vi "C-885 Test Panel.vi"() -> ()   [LabVIEW 2016]
uses:
  PI GCS2 DLL/PI_GCS2_DLL_x64.dll
panel:
  in  "Set Point":dbl=0.1 format="%#_13g"
  out "Success":u32
  in  "stop":bool
  out "Positions 2":dbl[](array[numeric])
  out "Positions":dbl[](array[numeric])
  out "On Target?":u32[](array[numeric])
  out "Axes Refed":u32[](array[numeric])
  out "Axes ON?":u32[](array[numeric])
  in  "Axes":string[](array[string])
  out "USB Connection Error":bool
  out "C-885 Found":bool
  out "Number Connected":i32
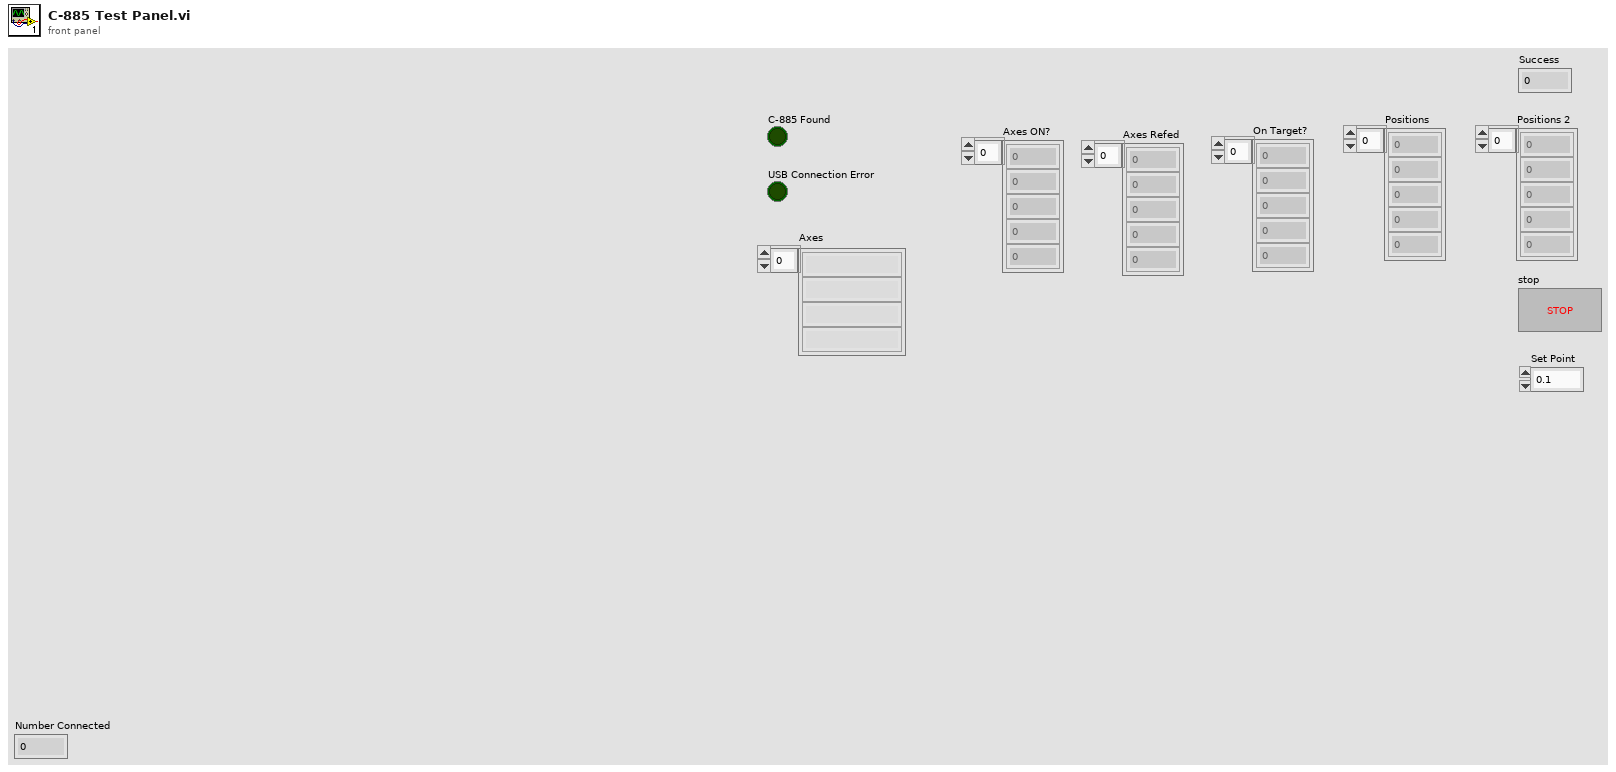
[diagram p1: front panel]
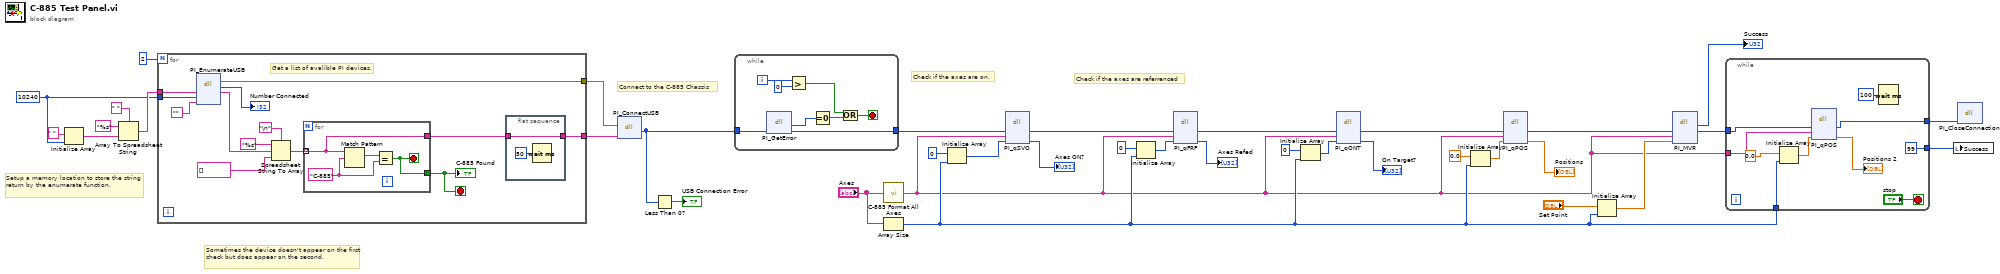
[diagram p0: block diagram]
diagram:
  w32 = 10240 ("dimension size")
  # "Check if the axes are referrenced"
  # "Check if the axes are on."
  # "Setup a memory location to store the string return by the enumerate function."
  # "Connect to the C-885 Chassis"
  # "Sometimes the device doesn't appear on the first check but does appear on the second."
  n1 = Initialize Array(" ", w32) -> (w36:string[])
  n2 = Array To Spreadsheet String(delimiter (Tab)=" ", array=w36, 3:"%s" ("format string")) -> (spreadsheet string=w33:string)
  n3 = for {
    N: 2 -> [_]
    tunnel: w33 -> [w45]
    tunnel: w32 -> [w44]
    tunnel: [w40] -> w30
    tunnel: [w38] -> w29
    stop <- w39 stop-if-true
    # "Get a list of avalible PI devices."
    n4 = dll-call lib="C:/Users/George Sirinakis/Documents/Microscope-Control/Device Library/Stages/PI/PI GCS2 DLL/PI_GCS2_DLL_x64.dll" fn="PI_EnumerateUSB"("szBuffer"=w45, "iBufferSize"=w44, "szFilter"="") -> (error out=w38:errorcluster, "return type"=→"Number Connected":i32, "szBuffer"=w42:string)  [unwired: 5 in, 1 out]
    n5 = Spreadsheet String To Array(delimiter (Tab)="\n", format string="%s", spreadsheet string=w42, array type (2D Dbl)=string[] []) -> (array=w47:string[])
    n6 = for {
      tunnel: w47 -> [w54] mode=indexing
      tunnel: [w54] -> w41
      tunnel: [w53] -> w39
      stop <- w53 stop-if-true
      w55 = "C-885"
      n7 = Match Pattern(string=w54, regular expression=w55) -> (match substring=w56:string)  [unwired: 1 in, 3 out]
      n8 = Equal?(x=w56, y=w55) -> (x = y?=w53:bool)
    }
    "C-885 Found" <- w39
    n9 = flat-sequence {
      tunnel: w41 -> [w52]
      tunnel: [w52] -> w40
      frame #0 {
        n10 = Wait (ms)(milliseconds to wait=u32 50) -> ()  [unwired: 1 out]
      }
    }
  }
  n11 = dll-call lib="C:/Users/George Sirinakis/Documents/Microscope-Control/Device Library/Stages/PI/PI GCS2 DLL/PI_GCS2_DLL_x64.dll" fn="PI_ConnectUSB"(error in=w29, "szDescription"=w30) -> ("Device ID"=w27:i32)  [unwired: 3 in, 2 out]
  n12 = Less Than 0?(x=w27) -> (x < 0?=→"USB Connection Error":bool)
  n13 = while {
    tunnel: w27 -> [w64]
    tunnel: [w63] -> w24
    i -> [w61]
    stop <- w57 stop-if-true
    n14 = dll-call lib="C:/Users/George Sirinakis/Documents/Microscope-Control/Device Library/Stages/PI/PI GCS2 DLL/PI_GCS2_DLL_x64.dll" fn="PI_GetError"("Device ID"=w64) -> ("Error Code"=w62:i32, "Device ID"=w63:i32)  [unwired: 3 in, 2 out]
    n15 = Greater?(x=w61, y=0) -> (0:w58:bool)
    n16 = Equal To 0?(x=w62) -> (x = 0?=w59:bool)
    n17 = Compound Arithmetic op=OR(w58, w59) -> (w57:bool)
  }
  n18 = call "C-885 Format All Axes.vi"("All Axis Array"="Axes") -> ("All Axes String"=w2:string)  [unwired: 14 in]
  n19 = Array Size(array="Axes") -> (size(s)=w5:i32)
  n20 = Initialize Array(u32 0 ("element"), w5) -> (w26:u32[])
  n21 = dll-call lib="C:/Users/George Sirinakis/Documents/Microscope-Control/Device Library/Stages/PI/PI GCS2 DLL/PI_GCS2_DLL_x64.dll" fn="PI_qSVO"("Device ID"=w24, "szAxes"=w2, "pdValueArray"=w26) -> ("Device ID"=w18:i32, "pdValueArray"=→"Axes ON?":u32[])  [unwired: 5 in, 2 out]
  n22 = Initialize Array(u32 0 ("element"), w5) -> (w20:u32[])
  n23 = dll-call lib="C:/Users/George Sirinakis/Documents/Microscope-Control/Device Library/Stages/PI/PI GCS2 DLL/PI_GCS2_DLL_x64.dll" fn="PI_qFRF"("Device ID"=w18, "szAxes"=w2, "pdValueArray"=w20) -> ("Device ID"=w15:i32, "pdValueArray"=→"Axes Refed":u32[])  [unwired: 5 in, 2 out]
  n24 = Initialize Array(u32 0 ("element"), w5) -> (w16:u32[])
  n25 = dll-call lib="C:/Users/George Sirinakis/Documents/Microscope-Control/Device Library/Stages/PI/PI GCS2 DLL/PI_GCS2_DLL_x64.dll" fn="PI_qONT"("Device ID"=w15, "szAxes"=w2, "pdValueArray"=w16) -> ("Device ID"=w11:i32, "pdValueArray"=→"On Target?":u32[])  [unwired: 5 in, 2 out]
  n26 = Initialize Array(0.0 ("element"), w5) -> (w13:dbl[])
  n27 = dll-call lib="C:/Users/George Sirinakis/Documents/Microscope-Control/Device Library/Stages/PI/PI GCS2 DLL/PI_GCS2_DLL_x64.dll" fn="PI_qPOS"("Device ID"=w11, "szAxes"=w2, "pdValueArray"=w13) -> ("Device ID"=w9:i32, "pdValueArray"=→"Positions":dbl[])  [unwired: 5 in, 2 out]
  n28 = Initialize Array("Set Point", w5) -> (w7:dbl[])
  n29 = dll-call lib="C:/Users/George Sirinakis/Documents/Microscope-Control/Device Library/Stages/PI/PI GCS2 DLL/PI_GCS2_DLL_x64.dll" fn="PI_MVR"("Device ID"=w9, "szAxes"=w2, "pdValueArray"=w7) -> ("Success"=→"Success":u32, "Device ID"=w6:i32)  [unwired: 5 in, 2 out]
  n30 = while {
    tunnel: w6 -> [w71]
    tunnel: w5 -> [w70]
    tunnel: w2 -> [w67]
    tunnel: [w66] -> w4
    tunnel: [u32 99 ("milliseconds to wait")] -> w1
    stop <- "stop" stop-if-true
    n31 = Initialize Array(0.0 ("element"), w70) -> (w68:dbl[])
    n32 = dll-call lib="C:/Users/George Sirinakis/Documents/Microscope-Control/Device Library/Stages/PI/PI GCS2 DLL/PI_GCS2_DLL_x64.dll" fn="PI_qPOS"("Device ID"=w71, "szAxes"=w67, "pdValueArray"=w68) -> ("Device ID"=w66:i32, "pdValueArray"=→"Positions 2":dbl[])  [unwired: 5 in, 2 out]
    n33 = Wait (ms)(milliseconds to wait=u32 100) -> ()  [unwired: 1 out]
  }
  n34 = local write "Success"(w1) -> ()
  n35 = dll-call lib="C:/Users/George Sirinakis/Documents/Microscope-Control/Device Library/Stages/PI/PI GCS2 DLL/PI_GCS2_DLL_x64.dll" fn="PI_CloseConnection"("Device ID"=w4) -> ()  [unwired: 5 in, 2 out]
